vi "Check Display Window.vi"(8 "Error In (no error)":errorcluster, 10 "Display Window (1)":i32=1, 11 "VISA Resource Name":refnum<visa-resource-name>) -> (0 "Error Out":errorcluster, 1 "Window Array":i32[](array[numeric]), 2 "Display Window Check":bool, 3 "VISA Resource Name Out":refnum<visa-resource-name>)   [LabVIEW 2018, in "Agilent PNA Series.lvlib"]
doc: "This VI checks that the display window number is valid for the selected channel."
uses:
  Agilent PNA Series.lvlib
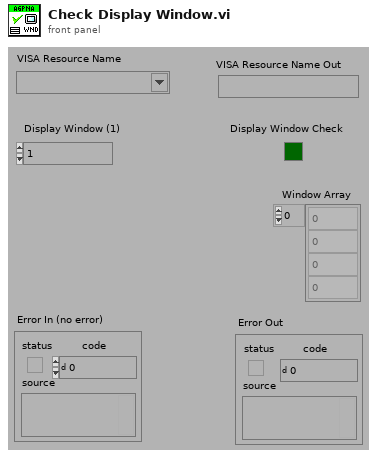
[diagram p1: front panel]
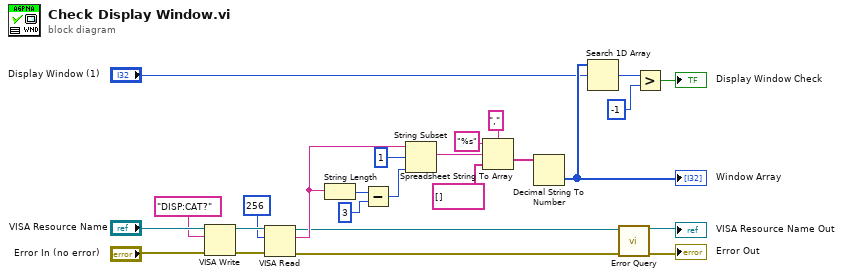
[diagram p0: block diagram]
diagram:
  n1 = VISA Write(VISA resource name="VISA Resource Name", write buffer="DISP:CAT?" ("format string"), error in (no error)="Error In (no error)") -> (VISA resource name out=w24:refnum<visa-resource-name>, error out=w23:errorcluster)  [unwired: 1 out]
  n2 = VISA Read(VISA resource name=w24, byte count=u32 256 ("byte count (0)"), error in (no error)=w23) -> (VISA resource name out=w4:refnum<visa-resource-name>, read buffer=w12:string, error out=w3:errorcluster)  [unwired: 1 out]
  n3 = String Length(string=w12) -> (length=w15:i32)
  n4 = Subtract(x=w15, y=3) -> (x-y=w13:i32)
  n5 = String Subset(string=w12, offset (0)=1, length (rest)=w13) -> (substring=w17:string)
  n6 = Spreadsheet String To Array(delimiter (Tab)=",", format string="%s", spreadsheet string=w17, array type (2D Dbl)=string[] []) -> (array=w11:string[])
  n7 = Decimal String To Number(string=w11) -> (number=w10:i32[])  [unwired: 2 in, 1 out]
  "Window Array" <- w10
  n8 = Search 1D Array(1D array=w10, element="Display Window (1)") -> (index of element=w8:i32)  [unwired: 1 in]
  n9 = call "Error Query.vi"("VISA Resource Name"=w4, "error in (no error)"=w3) -> ("VISA Resource Name Out"=→"VISA Resource Name Out":refnum<visa-resource-name>, "error out"=→"Error Out":errorcluster)  [unwired: 10 in, 2 out]
  n10 = Greater?(x=w8, y=-1) -> (0:→"Display Window Check":bool)
